vi "set_data_for_this_device.vi"(8 "error in (no error)":errorcluster, 10 "data":dbl[][](array[numeric]), 11 "DAQmxWriteSignals in":refnum<class "SignalWriterMM140725DAQmx.lvclass">) -> (0 "error out":errorcluster, 3 "DAQmxWriteSignals out":refnum<class "SignalWriterMM140725DAQmx.lvclass">)   [LabVIEW 2010, in "SignalWriterMM140725DAQmx.lvclass"]
uses:
  SignalWriterMM140725DAQmx.lvclass
  common/enumerations/functional_global_action_enum.ctl
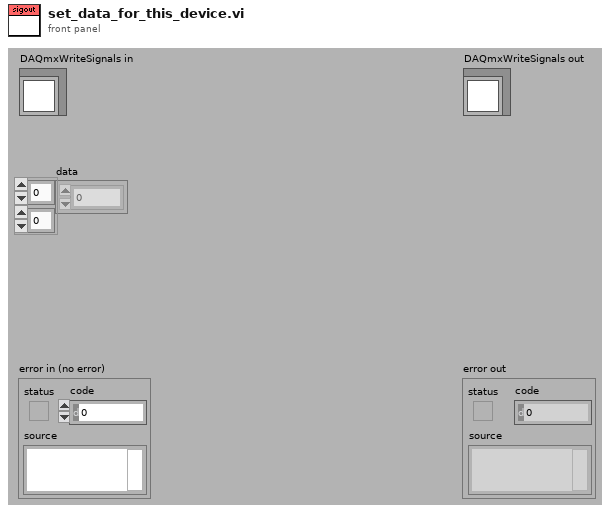
[diagram p1: front panel]
types:
  T1 = typedef "functional_global_action_enum.ctl" = enum16{"get", "set", "reset"}
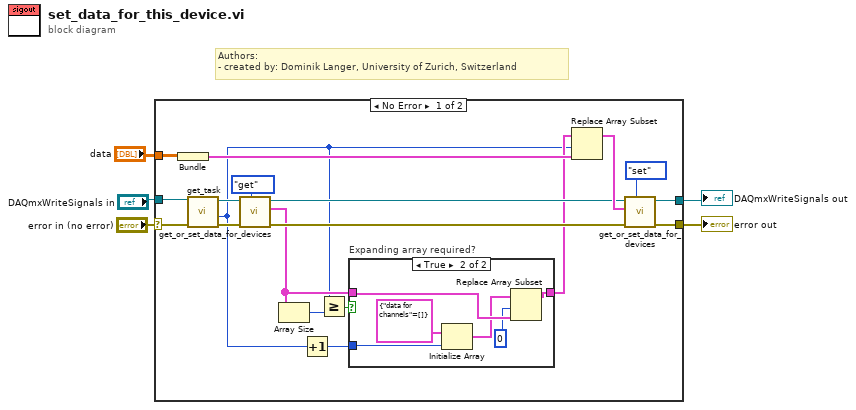
[diagram p0: block diagram]
diagram:
  # "Authors: \n- created by: Dominik Langer, University of Zurich, Switzerland"
  n1 = case shown="No Error" "error in (no error)" {
    selector: "error in (no error)" -> [w24 w33]
    tunnel: [w17 w33] -> w1
    tunnel: [w13 w32] -> w5
    tunnel: "DAQmxWriteSignals in" -> [w23 w32]
    tunnel: "data" -> [w21 _]
    frame No Error {
      n2 = Bundle("data"=w21) -> (w22:cluster{"data":dbl[][]})  [unwired: 1 in]
      n3 = call-dynamic "get_task.vi"("error in (no error)"=w24, "DAQmxWriteSignals in"=w23) -> ("error out"=w20:errorcluster, "index"=w6:i32, "DAQmxWriteSignals out"=w19:refnum<class "SignalWriterMM140725DAQmx.lvclass">)  [unwired: 7 out]
      n4 = call-dynamic "get_or_set_data_for_devices.vi"("action"=functional_global_action_enum."get", "error in (no error)"=w20, "DAQmxWriteSignals in"=w19) -> ("error out"=w16:errorcluster, "data for devices out"=w8:cluster{"data for channels":dbl[][]}[], "DAQmxWriteSignals out"=w14:refnum<class "SignalWriterMM140725DAQmx.lvclass">)  [unwired: 1 in, 5 out]
      n5 = Array Size(array=w8) -> (size(s)=w11:i32)
      n6 = Increment(x=w6) -> (x+1=w7:i32)
      n7 = Greater Or Equal?(x=w6, y=w11) -> (x >= y?=w9:bool)
      n8 = case "Expanding array required?" shown="True" w9 {
        tunnel: w7 -> [_ w31]
        tunnel: w8 -> [w25 w29]
        tunnel: [w25 w27] -> w10
        frame False {
        }
        frame True {
          n9 = Initialize Array(cluster{"data for channels":dbl[][]} {"data for channels"=[]} ("device"), w31) -> (w26:cluster{"data for channels":dbl[][]}[])
          n10 = Replace Array Subset(array=w26, new element=w29, index=0) -> (w27:cluster{"data for channels":dbl[][]}[])
        }
      }
      n11 = Replace Array Subset(array=w10, new element=w22, index=w6) -> (w15:cluster{"data for channels":dbl[][]}[])
      n12 = call-dynamic "get_or_set_data_for_devices.vi"("action"=functional_global_action_enum."set", "error in (no error)"=w16, "data for devices in"=w15, "DAQmxWriteSignals in"=w14) -> ("error out"=w17:errorcluster, "DAQmxWriteSignals out"=w13:refnum<class "SignalWriterMM140725DAQmx.lvclass">)  [unwired: 6 out]
    }
    frame Error {
    }
  }
  "error out" <- w1
  "DAQmxWriteSignals out" <- w5
